vi "plot gaussian wave.vi"() -> (3 "Array":dbl[](array[numeric]))   [LabVIEW 2020]
panel:
  out "Waveform Graph":dbl[](graph)
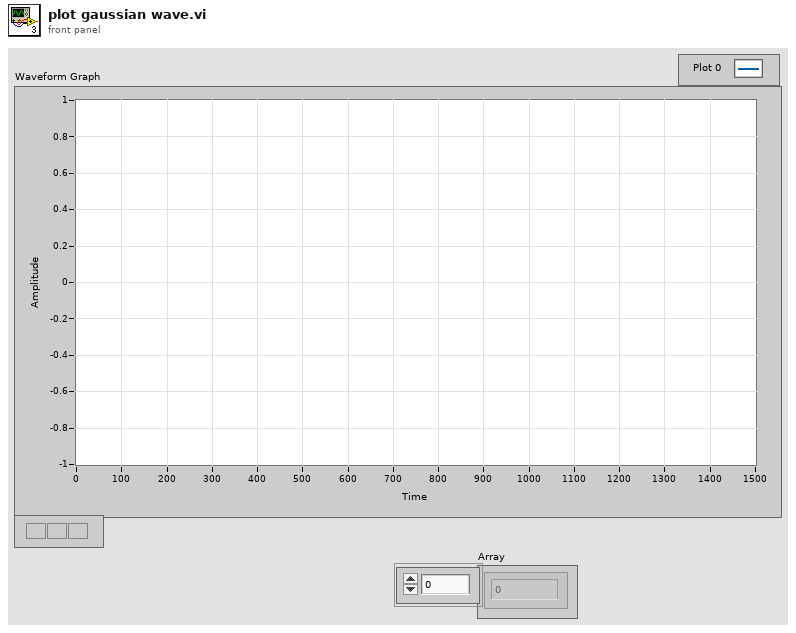
[diagram p1: front panel]
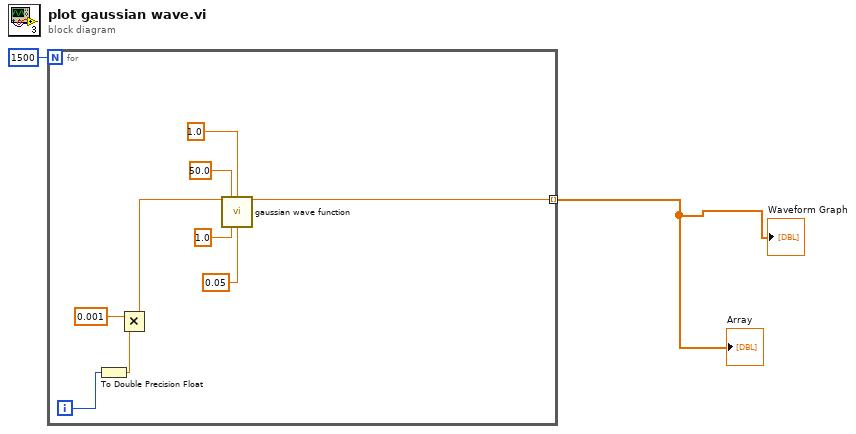
[diagram p0: block diagram]
diagram:
  n1 = for {
    N: 1500 -> [_]
    tunnel: [w5] -> w1 mode=indexing
    i -> [w7]
    n2 = To Double Precision Float(number=w7) -> (double precision float=w6:dbl)
    n3 = Multiply(x=0.001, y=w6) -> (x*y=w4:dbl)
    n4 = call "gaussian wave function.vi"("t us"=w4, "f MHz"=50.0, "phase0 pi"=1.0, "peak position us"=1.0, "sd us"=0.05) -> ("Result"=w5:dbl)  [unwired: 10 in]
  }
  "Waveform Graph" <- w1
  "Array" <- w1
